vi "Handle Error.vi"(8 "error in (no error)":errorcluster, 11 "Device in":refnum<class "Device.lvclass">) -> (0 "error out":errorcluster, 2 "stop actor?":bool=TRUE, 3 "Device out":refnum<class "Device.lvclass">)   [LabVIEW 2023, in "Device.lvlib" / "Device.lvclass"]
doc: "(<B>Filename</B>: Actor Framework.lvlib:Actor.lvclass:Handle Error.vi)\n\nDefines how the actor handles an error that occurred while processing a message.\n\nBy default, this method does nothing except stop the actor. This method also treats error code 43 (coming from <B>error in</B>) as a sign that the actor shut down normally. In this situation, the Handle Error method does not return the error on <B>error out</B>, meaning the actor's caller will not receive it. All other error codes will be returned on <B>error out</B>.\n\nA descendant class may override this method to change this behavior."
uses:
  Device.lvclass
  <vilib>/ActorFramework/Actor/Actor.lvclass/Actor.ctl
  Device.lvclass/Device.ctl
  Application Messages/Automation_TaskFailed Msg/Automation_TaskFailed Msg.lvclass/Automation_TaskFailed Msg.ctl
  <vilib>/ActorFramework/Message Enqueuer/Message Enqueuer.lvclass/Message Enqueuer.ctl
  <vilib>/ActorFramework/Message Enqueuer/Enqueue.vi
  Application Messages/Automation_TaskFailed Msg/Automation_TaskFailed Msg.lvclass
  <vilib>/ActorFramework/Message Priority Queue/Priority Enqueue.vi
  <vilib>/ActorFramework/Actor/Actor.lvclass
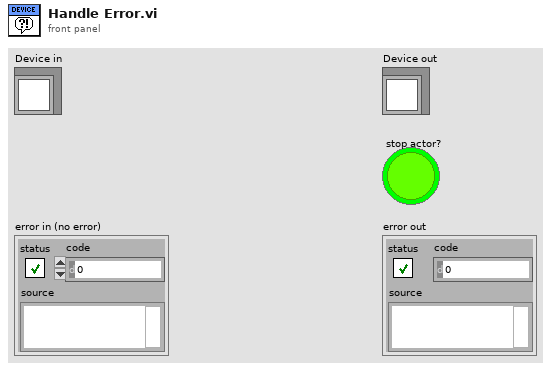
[diagram p1: front panel]
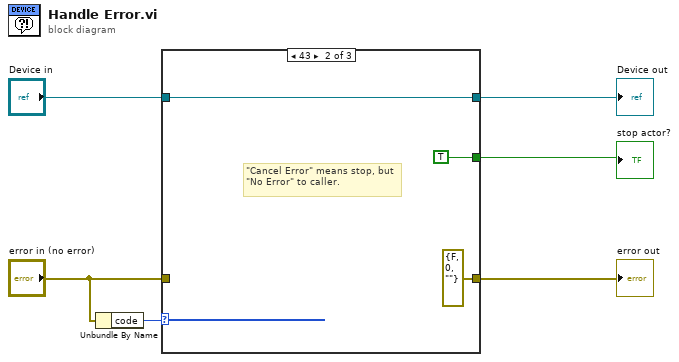
[diagram p0: block diagram]
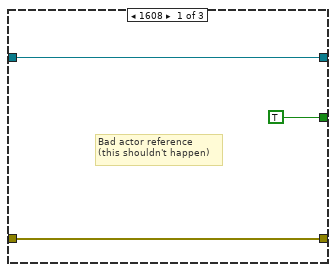
[diagram p2: hidden frame]
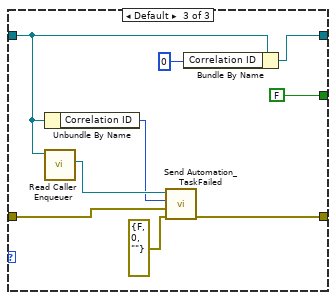
[diagram p3: hidden frame]
diagram:
  n1 = Unbundle By Name("error in (no error)") -> ("code"=w5:i32)
  n2 = case shown="43" w5 {
    tunnel: [w8 errorcluster {"status"=FALSE, "code"=0, "source"=""} ("error out") w16] -> w2
    tunnel: "error in (no error)" -> [w8 _ w15]
    tunnel: "Device in" -> [w9 w12 w19]
    tunnel: [w9 w12 w18] -> w3
    tunnel: [TRUE ("stop actor?") TRUE ("stop actor?") FALSE ("stop actor?")] -> w1
    frame 1608 {
      # "Bad actor reference\n(this shouldn't happen)"
    }
    frame 43 {
      # "\"Cancel Error\" means stop, but \"No Error\" to caller."
    }
    frame Default {
      n3 = Unbundle By Name(w19) -> ("Correlation ID"=w20:u32)
      n4 = call <vilib>:"Read Caller Enqueuer.vi"("Actor"=w19) -> ("Caller Enqueuer"=w21:refnum<class "Message Enqueuer.lvclass">)  [unwired: 10 in]
      n5 = call "Send Automation_TaskFailed.vi"("error in (no error)"=errorcluster {"status"=FALSE, "code"=0, "source"=""} ("error constant"), "device error"=w15, "Correlation ID"=w20, "Message Enqueuer"=w21) -> ("error out"=w16:errorcluster)  [unwired: 6 in, 1 out]
      n6 = Bundle By Name(cluster=w19, "Correlation ID"=u32 0) -> (w18:refnum<class "Device.lvclass">)
    }
  }
  "Device out" <- w3
  "error out" <- w2
  "stop actor?" <- w1
